vi "UCluClu Error Append Call Chain.vi"(3 "error in (no error)":errorcluster) -> (0 "error out":errorcluster)   [LabVIEW 2011]
doc: "Appends the calling chain onto the message in the source block in the error cluser. The first element of the calling chain is stripped off, so this VI's name will not WARNING: This vi has no code to determine if an error is present or not. It will append the entire call chain even if there is no error present."
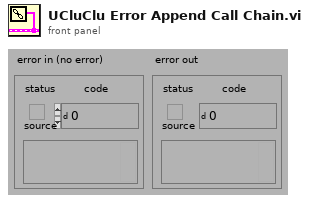
[diagram p1: front panel]
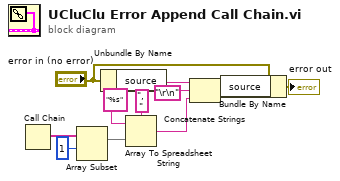
[diagram p0: block diagram]
diagram:
  n1 = Call Chain() -> (call chain=w10:string[])
  n2 = Array Subset(array=w10, index=1) -> (w8:string[])  [unwired: 1 in]
  n3 = Unbundle By Name("error in (no error)") -> ("source"=w11:string)
  n4 = Array To Spreadsheet String(delimiter (Tab)=", ", array=w8, 3:"%s" ("format string")) -> (spreadsheet string=w2:string)
  n5 = Concatenate Strings(w11, "\r\n", w2) -> (w5:string)
  n6 = Bundle By Name(cluster="error in (no error)", "source"=w5) -> (→"error out":errorcluster)
